vi "TraverseCtrl.vi"(1 "Input":cluster{"Name":string, "Ctrl":refnum<vi>}[](array[cluster]), 2 "Prefix":string, 3 "Ctrl Reference":refnum<vi>) -> (0 "Output":cluster{"Name":string, "Ctrl":refnum<vi>}[](array[cluster]))   [LabVIEW 2014]
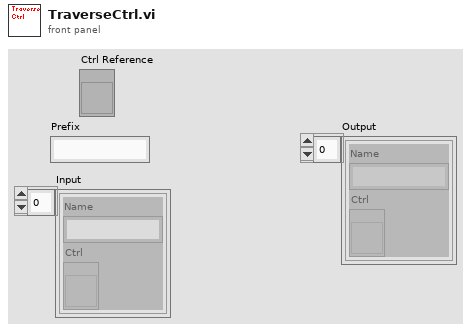
[diagram p1: front panel]
types:
  T1 = cluster{"Name":string, "Ctrl Reference":refnum<vi>}[]
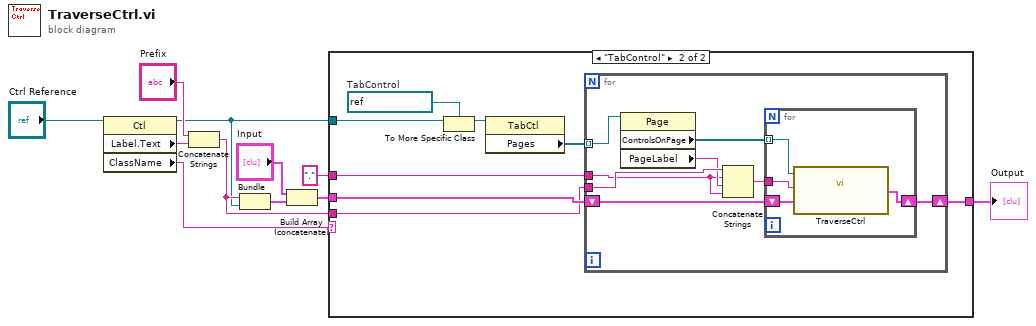
[diagram p0: block diagram]
diagram:
  n1 = property class="Ctl"(reference="Ctrl Reference") -> (reference out=w2:refnum<vi>, "Label.Text"=w8:string, "ClassName"=w11:string)  [unwired: 1 in, 1 out]
  n2 = Concatenate Strings("Prefix", w8) -> (w3:string)
  n3 = Bundle(w3, "Ctrl Reference"=w2) -> (w6:cluster{string, "Ctrl Reference":refnum<vi>})  [unwired: 1 in]
  n4 = Build Array (concatenate)("Input", w6) -> (w4:T1)
  n5 = case shown="\"TabControl\"" w11 {
    tunnel: [w12 w17] -> w7
    tunnel: w4 -> [w12 w16]
    tunnel: w3 -> [_ w15]
    tunnel: w2 -> [_ w14]
    tunnel: "." ("string") -> [_ w13]
    frame Default {
    }
    frame "TabControl" {
      w20 = refnum<vi> refnum  # TabControl
      n6 = To More Specific Class(target class=w20, reference=w14) -> (specific class reference=w19:refnum<vi>)  [unwired: 1 in, 1 out]
      n7 = property class="TabCtl"(reference=w19) -> ("Pages"=w18:refnum<vi>[])  [unwired: 1 in, 2 out]
      n8 = for {
        tunnel: w18 -> [w28] mode=indexing
        tunnel: w15 -> [w26]
        shift-right: [w23] -> w17
        shift-left: w16 -> [w24]
        tunnel: w13 -> [w21]
        n9 = property class="Page"(reference=w28) -> ("ControlsOnPage"=w27:refnum<vi>[], "PageLabel"=w22:string)  [unwired: 1 in, 2 out]
        n10 = Concatenate Strings(w26, w21, w22, w21) -> (w25:string)
        n11 = for {
          tunnel: w27 -> [w32] mode=indexing
          tunnel: w25 -> [w31]
          shift-right: [w29] -> w23
          shift-left: w24 -> [w30]
          n12 = call "TraverseCtrl.vi"("Input"=w30, "Prefix"=w31, "Ctrl Reference"=w32) -> ("Output"=w29:cluster{"Name":string, "Ctrl":refnum<vi>}[])
        }
      }
    }
  }
  "Output" <- w7
